vi "Traverse_Space_Server.vi"(4 "Space File":path, 6 "Mode":T4(ring), 7 "Entire Space":T1=[{"Max"=15001.0, "Min"=12000.0}, {"Max"=1000.0, "Min"=-1000.0}, {"Max"=700.0, "Min"=0.0}] {"Min" format="%#.1f"; "Max" format="%#.1f"}, 8 "Probe Volume":T1=[{"Max"=0.0, "Min"=0.0}, {"Max"=250.0, "Min"=0.0}, {"Max"=15.0, "Min"=-15.0}] {"Min" format="%#.1f"; "Max" format="%#.1f"}, 9 "Exclude Array":T2[](array[typedef]) {"Sizes"."Min" format="%#.1f"; "Sizes"."Max" format="%#.1f"}, 10 "Traverse Name":string) -> (0 "Entire Space Out":T1=[{"Max"=15001.0, "Min"=12000.0}, {"Max"=1000.0, "Min"=-1000.0}, {"Max"=700.0, "Min"=0.0}] {"Min" format="%#.1f"; "Max" format="%#.1f"}, 1 "Probe Volume Out":T1=[{"Max"=15.0, "Min"=-15.0}, {"Max"=250.0, "Min"=0.0}, {"Max"=15.0, "Min"=-15.0}] {"Min" format="%#.1f"; "Max" format="%#.1f"}, 2 "Exclude Array Out":T2[](array[typedef])=[{"Sizes"=[{"Max"=15000.0, "Min"=0.0}, {"Max"=1000.0, "Min"=-1000.0}, {"Max"=300.0, "Min"=0.0}], "Name"="Roughness Elements", "Exclude Type"=enum."Allow only vertical moves"}, {"Sizes"=[{"Max"=17000.0, "Min"=16000.0}, {"Max"=200.0, "Min"=-200.0}, {"Max"=-50.0, "Min"=-250.0}], "Name"="B204", "Exclude Type"=enum."Exclude completely"}] {"Sizes"."Min" format="%#.1f"; "Sizes"."Max" format="%#.1f"}, 3 "Error Comments":string)   [LabVIEW 2011]
uses:
  Gen Trav/Route mapping/Exclude_cluster.ctl
  Gen Trav/Route mapping/Box_size.ctl
  Gen Trav/Route mapping/Exclusion_type.ctl
panel:
  in  "Integer":i32
  out "Channel Values":string[][](array[string])
  # "(Relative to measurement position)"
  # "(Relative to measurement position)"
  # "X                           Y                          Z"
  # "X                           Y                          Z"
  # "X                           Y                          Z"
  # "X                           Y                          Z"
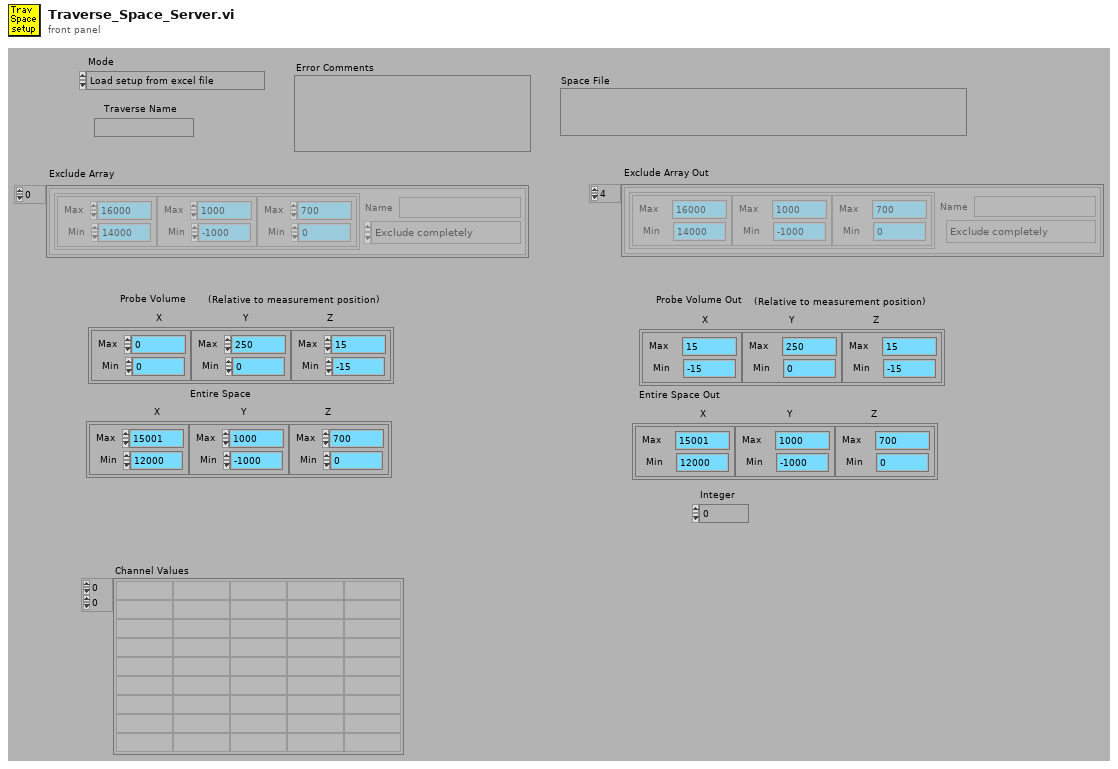
[diagram p1: front panel]
types:
  T1 = typedef "Box_size.ctl" = cluster{"Max":dbl, "Min":dbl}[]
  T2 = typedef "Exclude_cluster.ctl" = cluster{"Sizes":T1, "Name":string, "Exclude Type":T3}
  T3 = typedef "Exclusion_type.ctl" = enum16{"Exclude completely", "Allow only vertical moves"}
  T4 = enum16{"Load setup from excel file", "Save setup to excel file"}
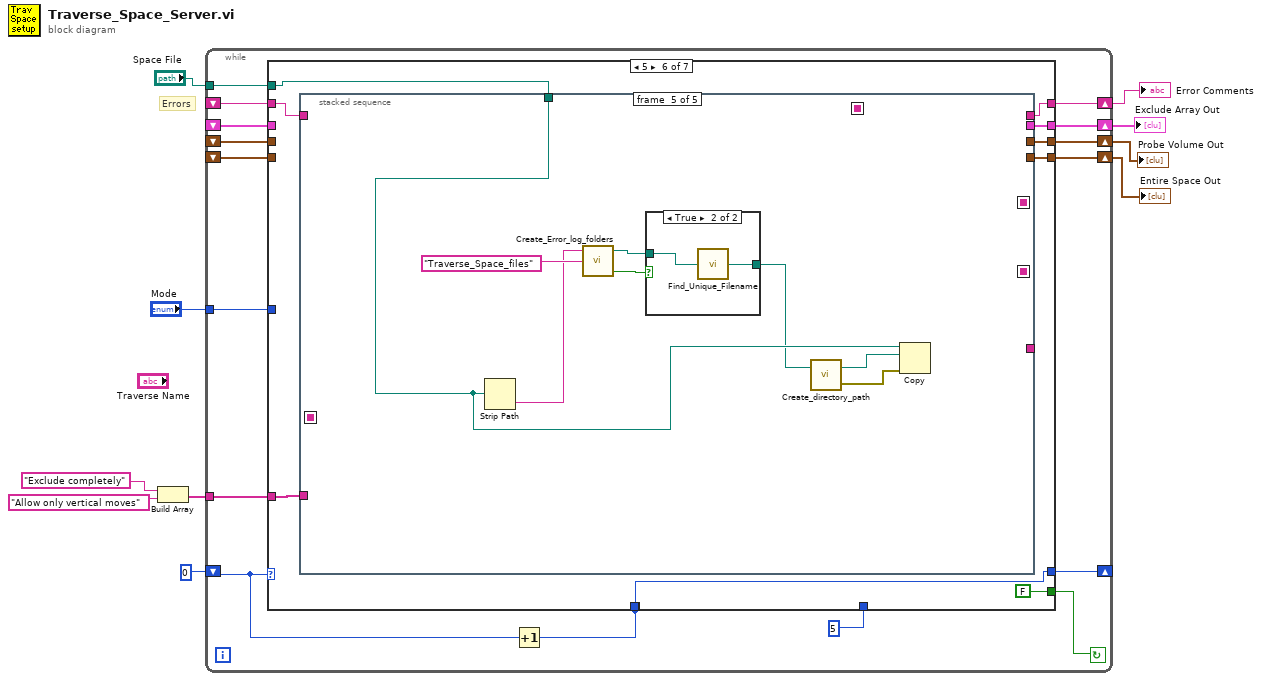
[diagram p0: block diagram]
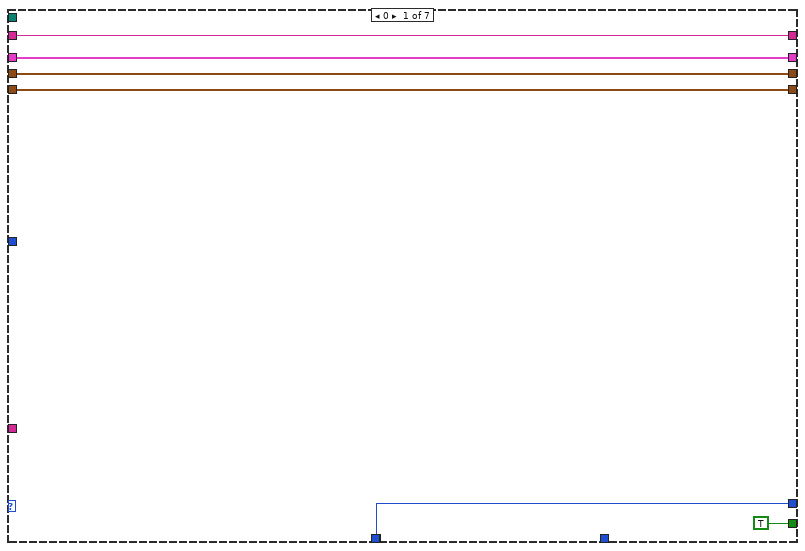
[diagram p2: hidden frame]
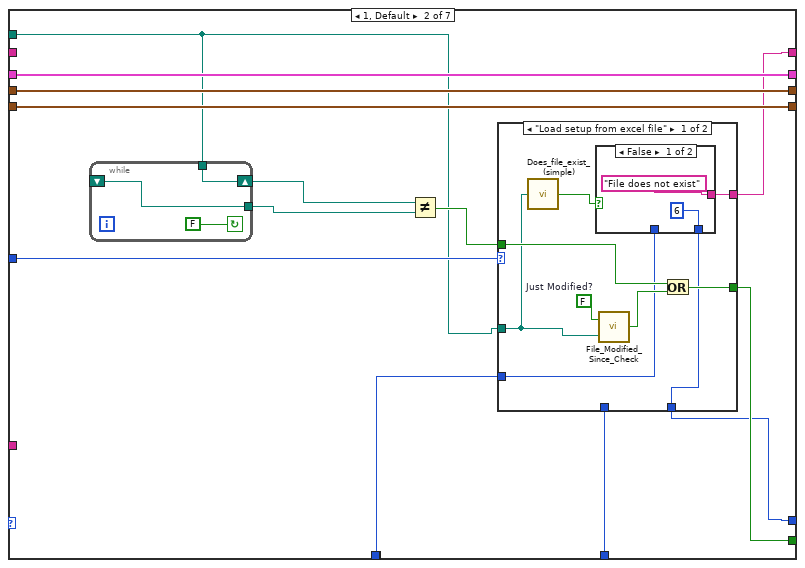
[diagram p3: hidden frame]
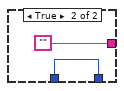
[diagram p4: hidden frame]
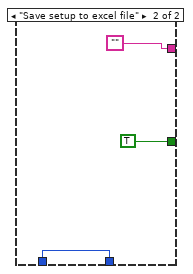
[diagram p5: hidden frame]
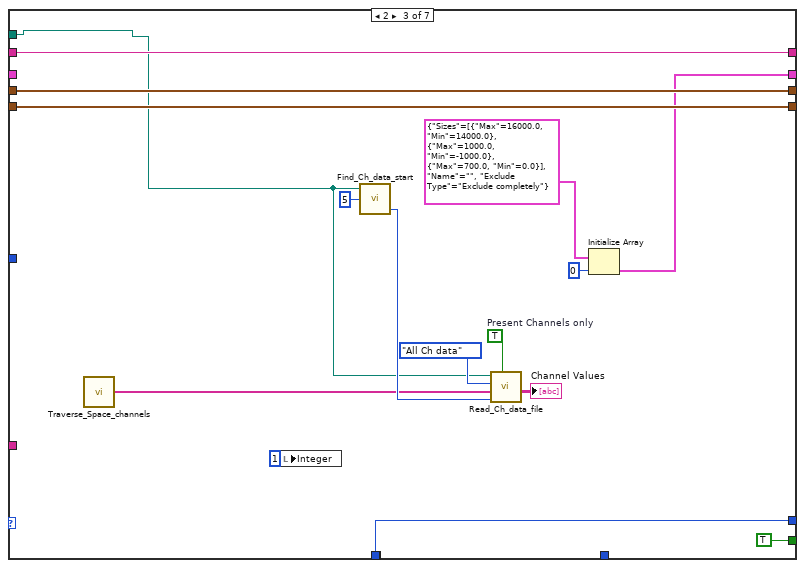
[diagram p6: hidden frame]
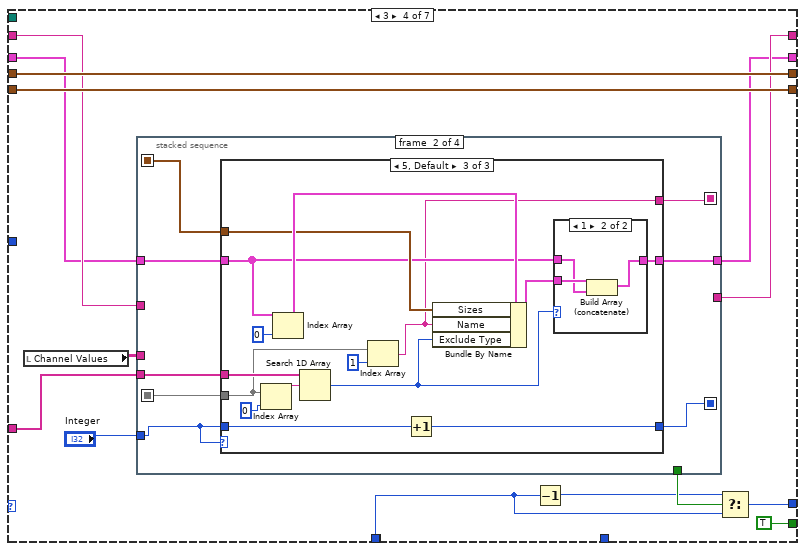
[diagram p7: hidden frame]
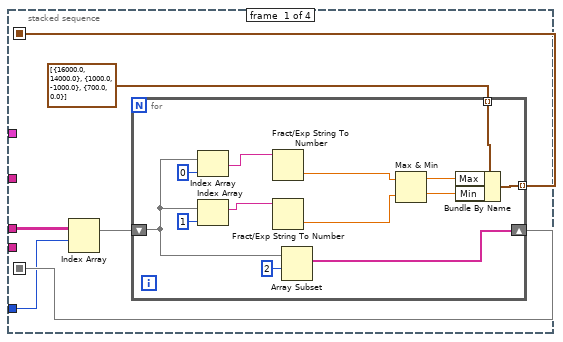
[diagram p8: hidden frame]
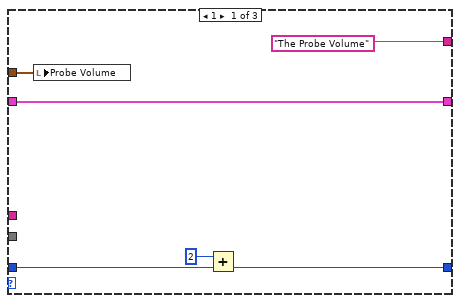
[diagram p9: hidden frame]
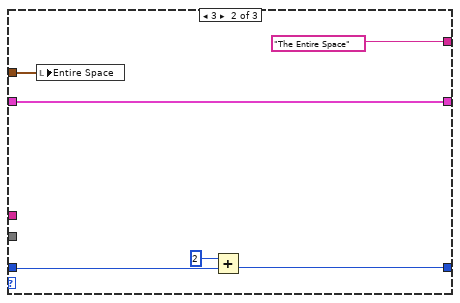
[diagram p10: hidden frame]
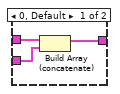
[diagram p11: hidden frame]
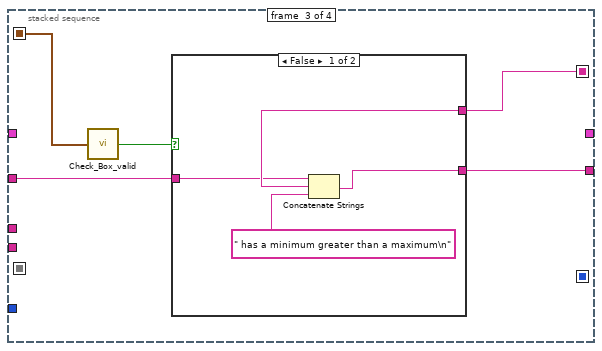
[diagram p12: hidden frame]
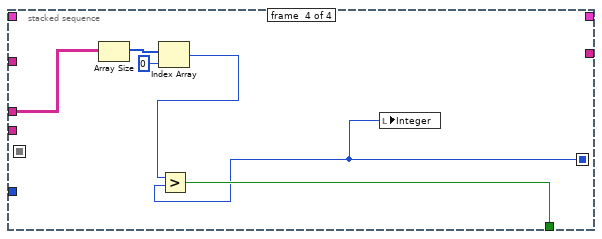
[diagram p14: hidden frame]
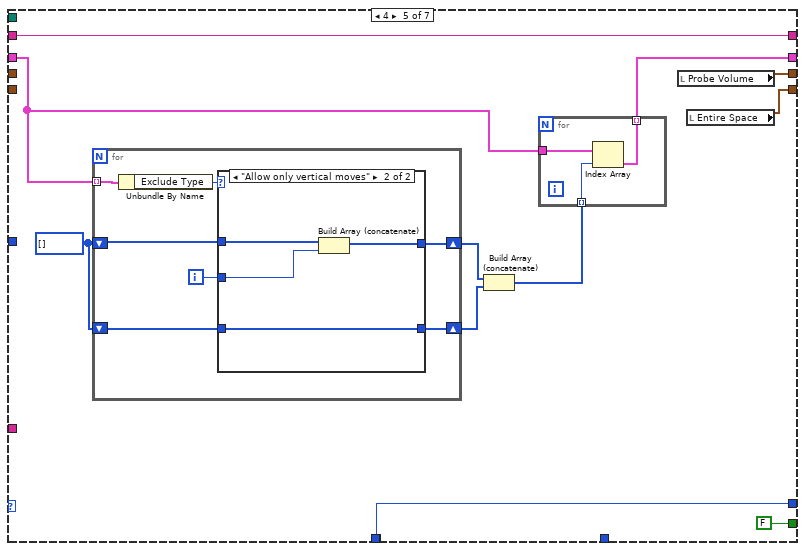
[diagram p15: hidden frame]
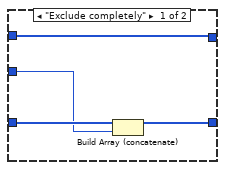
[diagram p16: hidden frame]
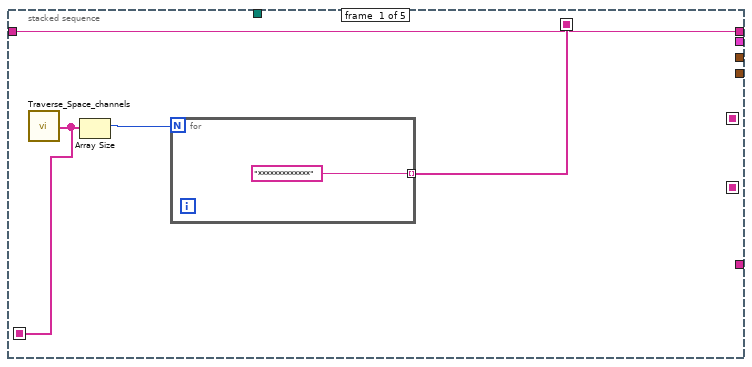
[diagram p17: hidden frame]
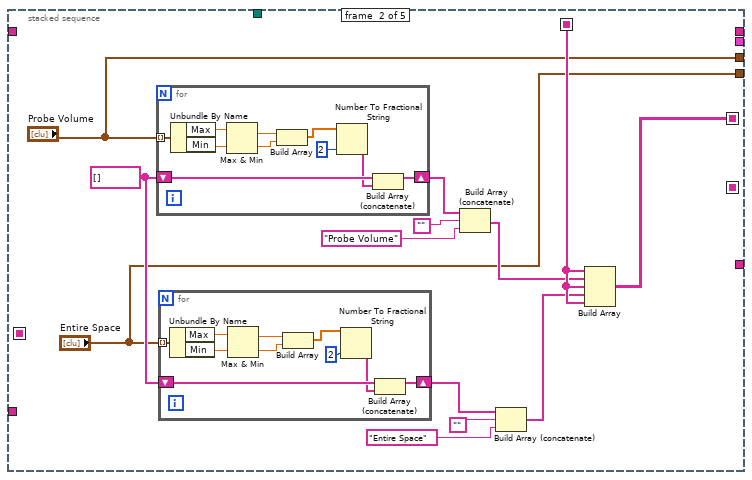
[diagram p18: hidden frame]
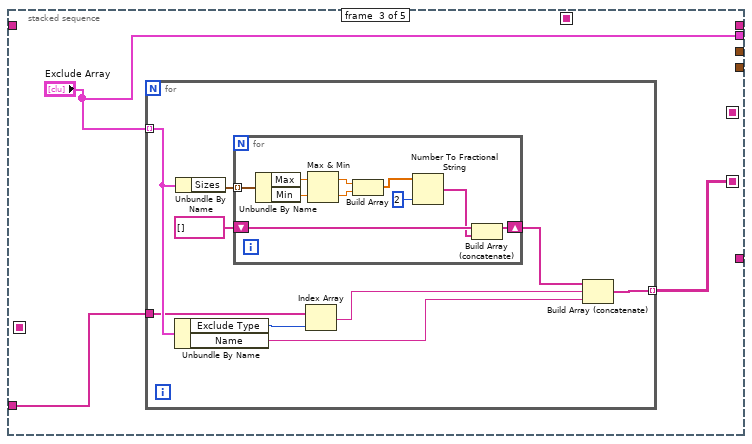
[diagram p19: hidden frame]
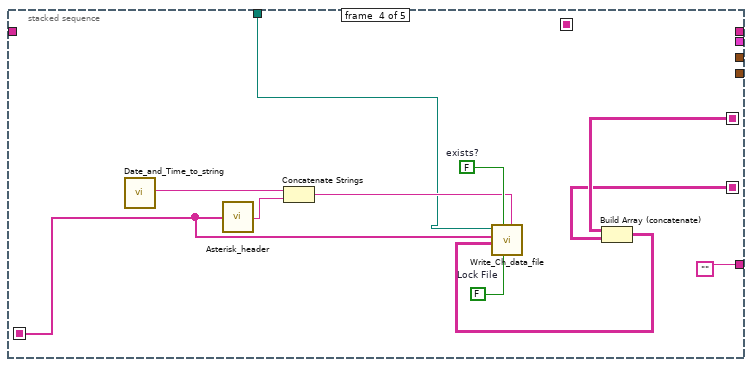
[diagram p20: hidden frame]
diagram:
  # "Errors"
  n1 = Build Array("Exclude completely", "Allow only vertical moves") -> (w3:string[])
  n2 = while {
    tunnel: w3 -> [w13]
    shift-left: _ -> [w16]
    shift-right: [w15] -> w2
    tunnel: "Mode" -> [w23]
    shift-left: _ -> [w19]
    shift-right: [w18] -> w7
    shift-left: _ -> [w21]
    shift-right: [w20] -> w8
    shift-left: _ -> [w22]
    shift-right: [w12] -> w9
    shift-left: 0 -> [w25]
    shift-right: [w24] -> _
    tunnel: "Space File" -> [w11]
    stop <- w26 continue-if-true
    n3 = Increment(x=w25) -> (x+1=w14:i32)
    n4 = case shown="5" w25 {
      tunnel: [TRUE w36 TRUE TRUE FALSE FALSE FALSE] -> w26
      tunnel: w14 -> [w28 w40 _ _ w179 w201 w295]
      tunnel: [w28 w34 w72 w83 w179 w201 w295] -> w24
      tunnel: w23 -> [_ w45 _ _ _ _ _]
      tunnel: w22 -> [w31 w43 _ w81 w172 _ _]
      tunnel: w21 -> [w30 w42 w75 w94 _ _ _]
      tunnel: [w30 w42 w75 w94 w178 w203 w292] -> w20
      tunnel: w19 -> [w29 w41 w74 w93 _ _ _]
      tunnel: [w29 w41 w74 w93 w177 w202 w292] -> w18
      tunnel: 5 -> [_ w39 _ _ _ _ _]
      tunnel: w16 -> [w32 _ w73 w88 w180 w205 w291]
      tunnel: [w32 w35 w73 w87 w180 w206 w291] -> w15
      tunnel: w14 -> [_ _ w72 w84 _ _ _]
      tunnel: w13 -> [_ _ _ w89 _ w207 _]
      tunnel: [w31 w43 w67 w82 w171 w204 T2[] [] ("Exclude Array")] -> w12
      tunnel: w11 -> [_ w33 w65 _ _ w200 _]
      frame 0 {
      }
      frame 1, Default {
        n5 = while {
          tunnel: [w48] -> w37
          shift-left: _ -> [w48]
          shift-right: [w46] -> w38
          tunnel: w33 -> [w46]
          stop <- FALSE continue-if-true
        }
        n6 = Not Equal?(x=w38, y=w37) -> (x != y?=w44:bool)
        n7 = case shown="\"Load setup from excel file\"" w45 {
          tunnel: w33 -> [w53 _]
          tunnel: w44 -> [w56 _]
          tunnel: [w55 TRUE] -> w36
          tunnel: w40 -> [w49 _]
          tunnel: [w50 w63] -> w34
          tunnel: w39 -> [_ w63]
          tunnel: [w51 ""] -> w35
          frame "Load setup from excel file" {
            w54 = FALSE  # Just Modified?
            n8 = call "Does_file_exist_(simple).vi"("Pathname"=w53) -> ("exists?"=w52:bool)
            n9 = case shown="False" w52 {
              tunnel: ["File does not exist" ""] -> w51
              tunnel: [6 ("f") w60] -> w50
              tunnel: w49 -> [_ w60]
              frame False {
              }
              frame True {
              }
            }
            n10 = call "File_Modified_Since_Check.vi"("Pathname"=w53, "Just Modified?"=w54) -> ("Modified?"=w57:bool)
            n11 = Or(x=w56, y=w57) -> (x .or. y?=w55:bool)
          }
          frame "Save setup to excel file" {
          }
        }
      }
      frame 2 {
        w77 = TRUE  # Present Channels only
        n12 = call "Traverse_Space_channels.vi"() -> ("Channel Names"=w66:string[])
        n13 = local write "Integer"(1 ("Integer")) -> ()
        n14 = call "Find_Ch_data_start.vi"("Approx No Of Columns"=5, "Filename"=w65) -> ("Start of read offset output"=w80:i32)  [unwired: 1 in, 2 out]
        n15 = call "Read_Ch_data_file.vi"("Present Channels only"=w77, "Start of read offset (chars.: 0)"=w80, "Present Channels"=w66, "Output"=enum16{"All Ch data", "The last few rows"}."All Ch data", "Filename"=w65) -> ("Channel Values"=→"Channel Values":string[][])  [unwired: 4 out]
        n16 = Initialize Array(T2 {"Sizes"=[{"Max"=16000.0, "Min"=14000.0}, {"Max"=1000.0, "Min"=-1000.0}, {"Max"=700.0, "Min"=0.0}], "Name"="", "Exclude Type"=enum."Exclude completely"} ("Cluster"), 0 ("Dimension Size")) -> (w67:T2[])
      }
      frame 3 {
        n17 = local read "Channel Values"() -> (w91:string[][])
        n18 = stacked-sequence {
          seq-local: [w95 _ _ _] -> [_ w121 w159 _]
          seq-local: [w97 _ _ _] -> [_ w116 _ _]
          seq-local: [_ w120 _ _] -> [_ _ w157 _]
          seq-local: [_ w114 _ _] -> [_ _ _ w165]
          tunnel: w91 -> [w100 _ _ w167]
          tunnel: "Integer" -> [w96 w115 _ _]
          tunnel: w88 -> [_ _ w156 _]
          tunnel: [_ _ w155 _] -> w87
          tunnel: [_ w119 _ _] -> w82
          tunnel: w81 -> [_ w118 _ _]
          tunnel: w89 -> [_ w117 _ _]
          tunnel: [_ _ _ w170] -> w86
          frame #0 {
            n19 = Index Array(array=w100, index (row)=w96) -> (element=w99:string[])  [unwired: 1 in]
            n20 = for {
              shift-right: [w111] -> w97
              shift-left: w99 -> [w110]
              tunnel: T1 [{"Max"=16000.0, "Min"=14000.0}, {"Max"=1000.0, "Min"=-1000.0}, {"Max"=700.0, "Min"=0.0}] ("Entire Space") -> [w106] mode=indexing
              tunnel: [w105] -> w95 mode=indexing
              n21 = Index Array(array=w110, index=0 ("Index")) -> (element=w108:string)
              n22 = Index Array(array=w110, index=1 ("Index")) -> (element=w107:string)
              n23 = Fract/Exp String To Number(string=w108) -> (number=w104:dbl)  [unwired: 4 out]
              n24 = Fract/Exp String To Number(string=w107) -> (number=w103:dbl)  [unwired: 4 out]
              n25 = Array Subset(array=w110, index=2 ("Array Index")) -> (w111:string[])  [unwired: 1 in]
              n26 = Max & Min(x=w104, y=w103) -> (max(x,y)=w102:dbl, min(x,y)=w101:dbl)
              n27 = Bundle By Name(cluster=w106, "Max"=w102, "Min"=w101) -> (w105:cluster{"Max":dbl, "Min":dbl})
            }
          }
          frame #1 {
            n28 = case shown="5, Default" w115 {
              tunnel: w121 -> [w122 w128 w146]
              tunnel: ["The Probe Volume" "The Entire Space" w137] -> w120
              tunnel: [w126 w132 w145] -> w119
              tunnel: w118 -> [w126 w132 w143]
              tunnel: w117 -> [_ _ w142]
              tunnel: w116 -> [_ _ w138]
              tunnel: w115 -> [w125 w130 w136]
              tunnel: [w123 w129 w135] -> w114
              frame 1 {
                n29 = local write "Probe Volume"(w122) -> ()
                n30 = Add(x=2, y=w125) -> (x+y=w123:i32)
              }
              frame 3 {
                n31 = local write "Entire Space"(w128) -> ()
                n32 = Add(x=2, y=w130) -> (x+y=w129:i32)
              }
              frame 5, Default {
                n33 = Index Array(array=w138, index=0 ("Index")) -> (element=w140:string)
                n34 = Index Array(array=w143, index=0 ("Index")) -> (element=w147:T2)
                n35 = Search 1D Array(1D array=w142, element=w140) -> (index of element=w134:i32)  [unwired: 1 out]
                n36 = Index Array(array=w138, index=1 ("Index")) -> (element=w137:string)
                n37 = Increment(x=w136) -> (x+1=w135:i32)
                n38 = Bundle By Name(cluster=w147, "Sizes"=w146, "Name"=w137, "Exclude Type"=w134) -> (w144:T2)
                n39 = case shown="1" w134 {
                  tunnel: [w151 w152] -> w145
                  tunnel: w144 -> [w150 w154]
                  tunnel: w143 -> [w149 w153]
                  frame 0, Default {
                    n40 = Build Array (concatenate)(w149, w150) -> (w151:T2[])
                  }
                  frame 1 {
                    n41 = Build Array (concatenate)(w154, w153) -> (w152:T2[])
                  }
                }
              }
            }
          }
          frame #2 {
            n42 = call "Check_Box_valid.vi"("Box to check"=w159) -> ("Valid Box"=w158:bool)
            n43 = case shown="False" w158 {
              tunnel: w157 -> [w162 _]
              tunnel: w156 -> [w161 w164]
              tunnel: [w160 w164] -> w155
              frame False {
                n44 = Concatenate Strings(w161, w162, " has a minimum greater than a maximum\n") -> (w160:string)
              }
              frame True {
              }
            }
          }
          frame #3 {
            n45 = Array Size(array=w167) -> (size(s)=w168:i32[])
            n46 = Index Array(array=w168, index=0 ("Index")) -> (element=w166:i32)
            n47 = Greater?(x=w166, y=w165) -> (0:w170:bool)
            n48 = local write "Integer"(w165) -> ()
          }
        }
        n49 = Decrement(x=w84) -> (x-1=w85:i32)
        n50 = Select(t=w85, s=w86, f=w84) -> (s? t:f=w83:i32)
      }
      frame 4 {
        w176 = i32[] []
        n51 = for {
          tunnel: w172 -> [w185] mode=indexing
          shift-right: [w189] -> w174
          shift-left: w176 -> [w190]
          shift-right: [w188] -> w175
          shift-left: w176 -> [w187]
          i -> [w186]
          n52 = Unbundle By Name(w185) -> ("Exclude Type"=w191:T3)
          n53 = case shown="\"Allow only vertical moves\"" w191 {
            tunnel: w190 -> [w193 w199]
            tunnel: [w193 w198] -> w189
            tunnel: [w194 w197] -> w188
            tunnel: w187 -> [w195 w197]
            tunnel: w186 -> [w192 w196]
            frame "Exclude completely" {
              n54 = Build Array (concatenate)(w195, w192) -> (w194:i32[])
            }
            frame "Allow only vertical moves" {
              n55 = Build Array (concatenate)(w199, w196) -> (w198:i32[])
            }
          }
        }
        n56 = Build Array (concatenate)(w174, w175) -> (w173:i32[])
        n57 = for {
          tunnel: w173 -> [w184] mode=indexing
          tunnel: w172 -> [w183]
          tunnel: [w182] -> w171 mode=indexing
          n58 = Index Array(array=w183, index=w184) -> (element=w182:T2)
        }
        n59 = local read "Probe Volume"() -> (w178:T1)
        n60 = local read "Entire Space"() -> (w177:T1)
      }
      frame 5 {
        n61 = stacked-sequence {
          seq-local: [_ _ w249 _ _] -> [_ _ _ w274 _]
          seq-local: [_ w225 _ _ _] -> [_ _ _ w275 _]
          seq-local: [w211 _ _ _ _] -> [_ w224 _ _ _]
          seq-local: [w209 _ _ _ _] -> [_ _ _ w270 _]
          tunnel: [_ _ _ "" _] -> _
          tunnel: w207 -> [_ _ w248 _ _]
          tunnel: [w210 _ _ _ _] -> w206
          tunnel: w205 -> [w210 _ _ _ _]
          tunnel: [_ _ "Exclude Array" _ _] -> w204
          tunnel: [_ "Probe Volume" _ _ _] -> w203
          tunnel: [_ "Entire Space" _ _ _] -> w202
          tunnel: w200 -> [_ _ _ w269 w284]
          frame #0 {
            n62 = call "Traverse_Space_channels.vi"() -> ("Channel Names"=w209:string[])
            n63 = Array Size(array=w209) -> (size(s)=w212:i32)
            n64 = for {
              N: w212 -> [_]
              tunnel: ["*************"] -> w211 mode=indexing
            }
          }
          frame #1 {
            w226 = string[] []
            n65 = for {
              tunnel: "Probe Volume" -> [w246] mode=indexing
              shift-right: [w241] -> w223
              shift-left: w226 -> [w243]
              n66 = Unbundle By Name(w246) -> ("Max"=w240:dbl, "Min"=w239:dbl)
              n67 = Max & Min(x=w240, y=w239) -> (max(x,y)=w238:dbl, min(x,y)=w237:dbl)
              n68 = Build Array(w238, w237) -> (w245:dbl[])
              n69 = Number To Fractional String(number=w245, precision (6)=i16 2) -> (F-format string=w242:string[])  [unwired: 2 out]
              n70 = Build Array (concatenate)(w243, w242) -> (w241:string[])
            }
            n71 = for {
              tunnel: "Entire Space" -> [w236] mode=indexing
              shift-right: [w231] -> w218
              shift-left: w226 -> [w233]
              n72 = Unbundle By Name(w236) -> ("Max"=w230:dbl, "Min"=w229:dbl)
              n73 = Max & Min(x=w230, y=w229) -> (max(x,y)=w228:dbl, min(x,y)=w227:dbl)
              n74 = Build Array(w228, w227) -> (w235:dbl[])
              n75 = Number To Fractional String(number=w235, precision (6)=i16 2) -> (F-format string=w232:string[])  [unwired: 2 out]
              n76 = Build Array (concatenate)(w233, w232) -> (w231:string[])
            }
            n77 = Build Array (concatenate)(w223, "", "Probe Volume" ("Input Element")) -> (w216:string[])
            n78 = Build Array (concatenate)(w218, "", "Entire Space" ("Input Element")) -> (w217:string[])
            n79 = Build Array(w224, w216, w224, w217, w224) -> (w225:string[][])
          }
          frame #2 {
            n80 = for {
              tunnel: "Exclude Array" -> [w256] mode=indexing
              tunnel: w248 -> [w254]
              tunnel: [w250] -> w249 mode=indexing
              n81 = Unbundle By Name(w256) -> ("Exclude Type"=w255:T3, "Name"=w251:string)
              n82 = Unbundle By Name(w256) -> ("Sizes"=w258:T1)
              n83 = for {
                tunnel: w258 -> [w268] mode=indexing
                shift-right: [w263] -> w253
                shift-left: string[] [] -> [w265]
                n84 = Unbundle By Name(w268) -> ("Max"=w262:dbl, "Min"=w261:dbl)
                n85 = Max & Min(x=w262, y=w261) -> (max(x,y)=w260:dbl, min(x,y)=w259:dbl)
                n86 = Build Array(w260, w259) -> (w267:dbl[])
                n87 = Number To Fractional String(number=w267, precision (6)=i16 2) -> (F-format string=w264:string[])  [unwired: 2 out]
                n88 = Build Array (concatenate)(w265, w264) -> (w263:string[])
              }
              n89 = Index Array(array=w254, index=w255) -> (element=w252:string)
              n90 = Build Array (concatenate)(w253, w252, w251) -> (w250:string[])
            }
          }
          frame #3 {
            w271 = FALSE  # Lock File
            w279 = FALSE  # exists?
            n91 = call "Date_and_Time_to_string.vi"() -> ("Date and time (spreadsheet)"=w276:string)
            n92 = call "Asterisk_header.vi"("Channel names"=w270) -> ("Header string"=w278:string)
            n93 = Concatenate Strings(w276, w278) -> (w277:string)
            n94 = Build Array (concatenate)(w275, w274) -> (w273:string[][])
            n95 = call "Write_Ch_data_file.vi"("Header string"=w277, "Lock File"=w271, "exists?"=w279, "Channel Values"=w273, "Channel names"=w270, "Filename"=w269) -> ()  [unwired: 2 in, 4 out]
          }
          frame #4 {
            n96 = Strip Path(path=w284) -> (name=w283:string)  [unwired: 1 out]
            n97 = call "Create_Error_log_folders.vi"("Log Folder"="Traverse_Space_files", "Log Filename"=w283) -> ("exists?"=w286:bool, "Local Log File"=w285:path)  [unwired: 1 in, 1 out]
            n98 = case shown="True" w286 {
              tunnel: [w288 w290] -> w282
              tunnel: w285 -> [w288 w289]
              frame False {
              }
              frame True {
                n99 = call "Find_Unique_Filename.vi"("Path In"=w289) -> ("Unique Path Out"=w290:path)  [unwired: 1 in, 1 out]
              }
            }
            n100 = call "Create_directory_path.vi"("Path name"=w282) -> ("error out"=w280:errorcluster, "Path name Out"=w281:path)  [unwired: 1 in]
            n101 = Copy(8:w280, 10:w281, 11:w284) -> ()  [unwired: 5 out]
          }
        }
      }
      frame 6 {
        w292 = T1 [] ("Probe Volume")
      }
    }
  }
  "Error Comments" <- w2
  "Probe Volume Out" <- w8
  "Entire Space Out" <- w7
  "Exclude Array Out" <- w9
